vi "ISX3_Cmd_GetDeviceId.vi"() -> (0 "DeviceID-Cmd":u8[](array[numeric]))   [LabVIEW 2012, in "Sciospec ISX3 Impedance Analyzer.lvlib"]
uses:
  Sciospec ISX3 Impedance Analyzer.lvlib
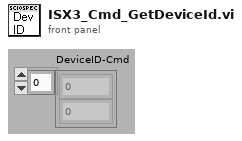
[diagram p1: front panel]
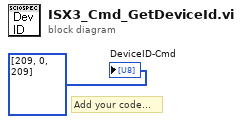
[diagram p0: block diagram]
diagram:
  # "Add your code..."
  "DeviceID-Cmd" <- u8[] [209, 0, 209]
